vi "Get Monitor Information.vi"(8 "error in":errorcluster) -> (0 "error out":errorcluster, 1 "Display info - Menu":string[](array[string]), 2 "no. Displays":i32, 3 "Display info":cluster{"Width":i16, "Height":i16}[](array[cluster]), 4 "Display:All Monitors":T1)   [LabVIEW 2014]
doc: "Provides information of all monitors that can be used as menu names/tags. \n\nIt places the primary monitor as the first element of the array.\n\nWindows: 0 is primary\nOS X: 1 is primary"
uses:
  <vilib>/Utility/miscctls.llb/LVAllMonitorsDisplayTypeDef.ctl
  <vilib>/Utility/miscctls.llb/LVRectTypeDef.ctl
panel:
  out "Display:Primary Workspace":T2
  out "Array":bool[](array[boolean])
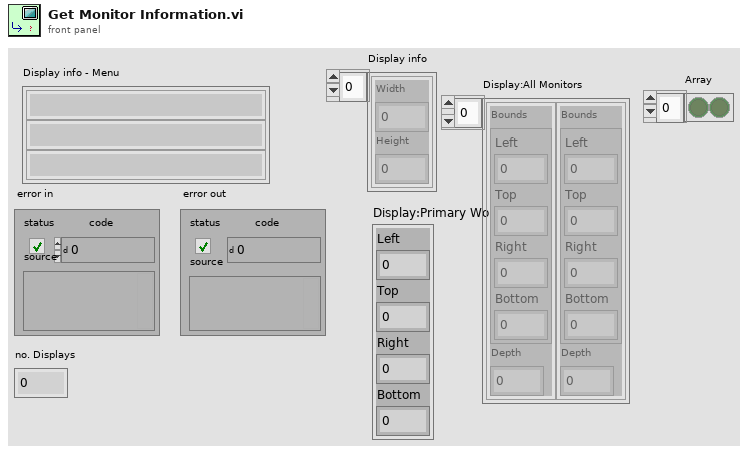
[diagram p1: front panel]
types:
  T1 = typedef "LVAllMonitorsDisplayTypeDef.ctl" = cluster{"Bounds":cluster{"Left":i16, "Top":i16, "Right":i16, "Bottom":i16}, "Depth":i16}[]
  T2 = typedef "LVRectTypeDef.ctl" = cluster{"Left":i16, "Top":i16, "Right":i16, "Bottom":i16}
  T3 = cluster{"Left":i16, "Top":i16, "Right":i16, "Bottom":i16}
  T4 = cluster{"Left":bool, "Top":bool, "Right":bool, "Bottom":bool}
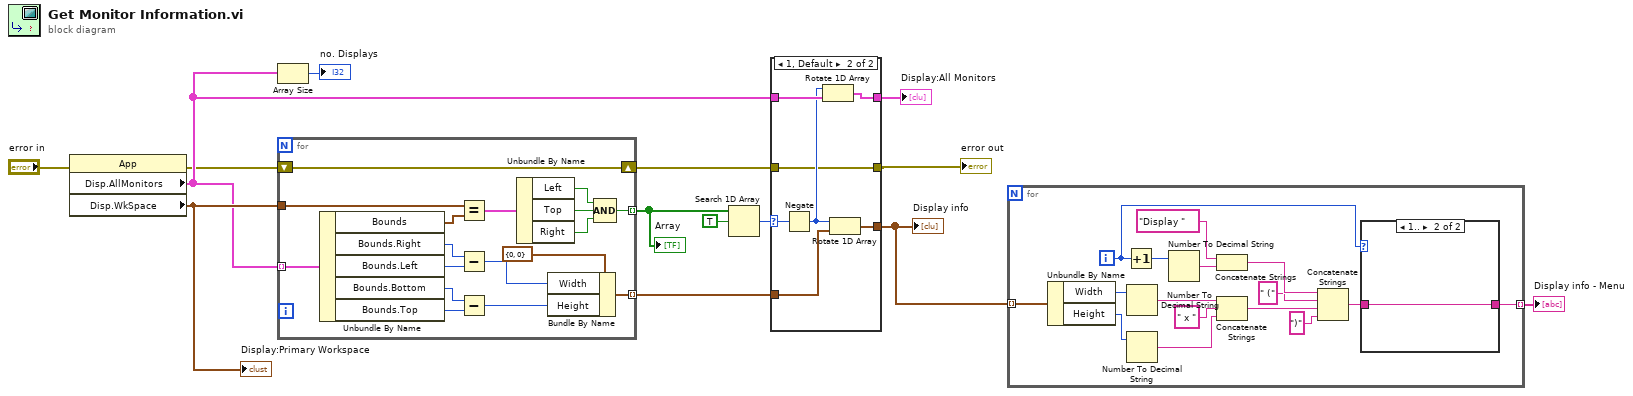
[diagram p0: block diagram]
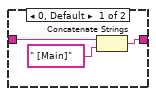
[diagram p3: hidden frame]
diagram:
  n1 = property class="App"(error in="error in") -> (error out=w2:errorcluster, "Disp.AllMonitors"=w5:T1, "Disp.WkSpace"=w6:T2)  [unwired: 1 in, 1 out]
  "Display:Primary Workspace" <- w6
  n2 = Array Size(array=w5) -> (size(s)=→"no. Displays":i32)
  n3 = for {
    tunnel: w5 -> [w31] mode=indexing
    tunnel: [w29] -> w10 mode=indexing
    tunnel: w6 -> [w21]
    tunnel: [w16] -> w12 mode=indexing
    shift-right: [w15] -> w3
    shift-left: w2 -> [w15]
    n4 = Unbundle By Name(w31) -> ("Bounds"=w22:T3, "Bounds.Right"=w28:i16, "Bounds.Left"=w27:i16, "Bounds.Bottom"=w25:i16, "Bounds.Top"=w26:i16)
    n5 = Equal?(x=w21, y=w22) -> (x = y?=w20:T4)
    n6 = Subtract(x=w28, y=w27) -> (x-y=w23:i16)
    n7 = Subtract(x=w25, y=w26) -> (x-y=w24:i16)
    n8 = Unbundle By Name(w20) -> ("Left"=w19:bool, "Top"=w18:bool, "Right"=w17:bool)
    n9 = Bundle By Name(cluster=cluster{"Width":i16, "Height":i16} {"Width"=0, "Height"=0}, "Width"=w23, "Height"=w24) -> (w29:cluster{"Width":i16, "Height":i16})
    n10 = Compound Arithmetic op=AND(w19, w18, w17) -> (w16:bool)
  }
  "Array" <- w12
  n11 = Search 1D Array(1D array=w12, element=TRUE) -> (index of element=w9:i32)  [unwired: 1 in]
  n12 = case shown="1, Default" w9 {
    selector: w9 -> [_ w40]
    tunnel: w10 -> [w34 w41]
    tunnel: [w34 w39] -> w8
    tunnel: w5 -> [w33 w37]
    tunnel: [w33 w38] -> w4
    tunnel: [w32 w35] -> w1
    tunnel: w3 -> [w32 w35]
    frame -1 {
    }
    frame 1, Default {
      n13 = Negate(x=w40) -> (-x=w36:i32)
      n14 = Rotate 1D Array(1:w37, 2:w36) -> (0:w38:T1)
      n15 = Rotate 1D Array(1:w41, 2:w36) -> (0:w39:cluster{"Width":i16, "Height":i16}[])
    }
  }
  "error out" <- w1
  "Display info" <- w8
  "Display:All Monitors" <- w4
  n16 = for {
    tunnel: w8 -> [w48] mode=indexing
    tunnel: [w42] -> w7 mode=indexing
    i -> [w44]
    n17 = Unbundle By Name(w48) -> ("Width"=w47:i16, "Height"=w46:i16)
    n18 = Increment(x=w44) -> (x+1=w49:i32)
    n19 = Number To Decimal String(number=w47) -> (decimal integer string=w56:string)  [unwired: 1 in]
    n20 = Number To Decimal String(number=w46) -> (decimal integer string=w54:string)  [unwired: 1 in]
    n21 = Number To Decimal String(number=w49) -> (decimal integer string=w57:string)  [unwired: 1 in]
    n22 = Concatenate Strings("Display " ("string"), w57) -> (w53:string)
    n23 = Concatenate Strings(w56, " x " ("string"), w54) -> (w51:string)
    n24 = Concatenate Strings(w53, " (" ("string"), w51, ")" ("string")) -> (w43:string)
    n25 = case shown="1.." w44 {
      tunnel: w43 -> [w60 w61]
      tunnel: [w58 w61] -> w42
      frame 0, Default {
        n26 = Concatenate Strings(w60, " [Main]" ("string")) -> (w58:string)
      }
      frame 1.. {
      }
    }
  }
  "Display info - Menu" <- w7
